vi "Semaphore.vi"() -> ()   [LabVIEW 2025]
panel:
  in  "Exit":bool
  in  "VISA resource name":refnum<visa-resource-name>
  in  "ON-OFF":bool
  in  "Enable ERROR Mod":bool
  in  "Timer ERROR":dbl
  in  "Timer ROSSO":dbl
  in  "Timer GIALLO":dbl
  in  "Timer VERDE":dbl
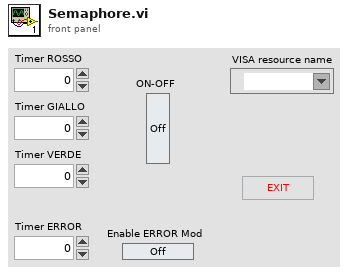
[diagram p1: front panel]
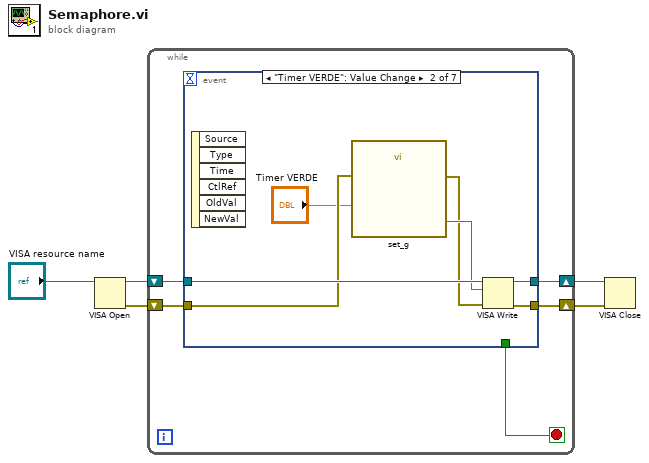
[diagram p0: block diagram]
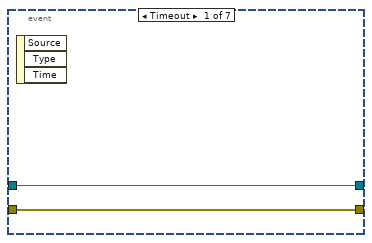
[diagram p2: hidden frame]
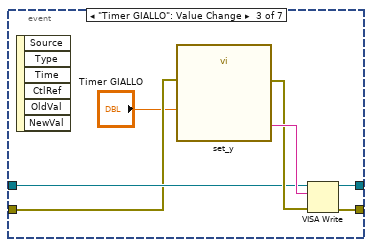
[diagram p3: hidden frame]
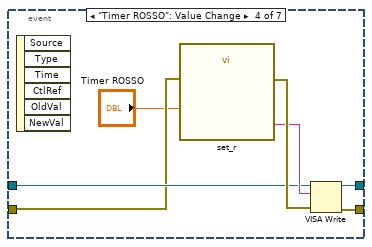
[diagram p4: hidden frame]
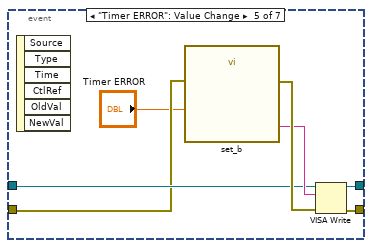
[diagram p5: hidden frame]
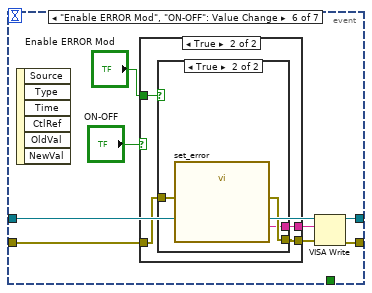
[diagram p6: hidden frame]
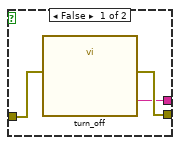
[diagram p7: hidden frame]
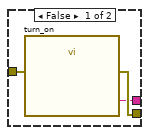
[diagram p8: hidden frame]
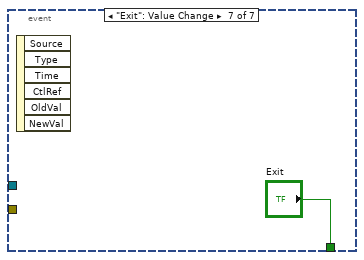
[diagram p9: hidden frame]
diagram:
  n1 = VISA Open(VISA resource name="VISA resource name") -> (VISA resource name=w3:refnum<visa-resource-name>, error out=w4:errorcluster)  [unwired: 4 in]
  n2 = while {
    shift-right: [w8] -> w2
    shift-left: w3 -> [w10]
    shift-right: [w7] -> w1
    shift-left: w4 -> [w9]
    stop <- w6 stop-if-true
    n3 = event shown="[1] \"Timer VERDE\": Value Change" {
      selector: _ -> [_ _ _ _ _ _ _]
      dyn-events: _ -> [_ _ _ _ _ _ _]
      timeout: _ -> [_ _ _ _ _ _ _]
      tunnel: w9 -> [w12 w16 w23 w30 w37 w44 _]
      tunnel: w10 -> [w11 w19 w24 w31 w38 w45 _]
      tunnel: [w11 w18 w22 w28 w35 w47 _] -> w8
      tunnel: [w12 w17 w21 w27 w34 w46 _] -> w7
      tunnel: [_ _ _ _ _ _ "Exit"] -> w6
      event Timeout {
        n4 = event-data() -> ()  [unwired: 1 in, 3 out]
      }
      event "Timer VERDE": Value Change {
        n5 = event-data() -> ()  [unwired: 1 in, 6 out]
        n6 = call "set_g"("timer"="Timer VERDE", "error in (no error)"=w16) -> ("Result"=w14:string, "error out"=w13:errorcluster)  [unwired: 12 in]
        n7 = VISA Write(VISA resource name=w19, write buffer=w14, error in (no error)=w13) -> (VISA resource name out=w18:refnum<visa-resource-name>, error out=w17:errorcluster)  [unwired: 1 out]
      }
      event "Timer GIALLO": Value Change {
        n8 = event-data() -> ()  [unwired: 1 in, 6 out]
        n9 = call "set_y"("timer"="Timer GIALLO", "error in (no error)"=w23) -> ("Result"=w26:string, "error out"=w25:errorcluster)  [unwired: 12 in]
        n10 = VISA Write(VISA resource name=w24, write buffer=w26, error in (no error)=w25) -> (VISA resource name out=w22:refnum<visa-resource-name>, error out=w21:errorcluster)  [unwired: 1 out]
      }
      event "Timer ROSSO": Value Change {
        n11 = event-data() -> ()  [unwired: 1 in, 6 out]
        n12 = call "set_r"("timer"="Timer ROSSO", "error in (no error)"=w30) -> ("Result"=w32:string, "error out"=w33:errorcluster)  [unwired: 12 in]
        n13 = VISA Write(VISA resource name=w31, write buffer=w32, error in (no error)=w33) -> (VISA resource name out=w28:refnum<visa-resource-name>, error out=w27:errorcluster)  [unwired: 1 out]
      }
      event "Timer ERROR": Value Change {
        n14 = event-data() -> ()  [unwired: 1 in, 6 out]
        n15 = call "set_b"("timer"="Timer ERROR", "error in (no error)"=w37) -> ("Result"=w39:string, "error out"=w40:errorcluster)  [unwired: 12 in]
        n16 = VISA Write(VISA resource name=w38, write buffer=w39, error in (no error)=w40) -> (VISA resource name out=w35:refnum<visa-resource-name>, error out=w34:errorcluster)  [unwired: 1 out]
      }
      event "Enable ERROR Mod", "ON-OFF": Value Change {
        n17 = event-data() -> ()  [unwired: 1 in, 6 out]
        n18 = case shown="True" "ON-OFF" {
          tunnel: w44 -> [w51 w54]
          tunnel: [w50 w53] -> w43
          tunnel: [w49 w52] -> w42
          tunnel: "Enable ERROR Mod" -> [_ w55]
          frame False {
            n19 = call "turn_off"("error in (no error)"=w51) -> ("Result"=w49:string, "error out"=w50:errorcluster)  [unwired: 13 in]
          }
          frame True {
            n20 = case shown="True" w55 {
              tunnel: w54 -> [w58 w61]
              tunnel: [w57 w60] -> w53
              tunnel: [w56 w59] -> w52
              frame False {
                n21 = call "turn_on"("error in (no error)"=w58) -> ("Result"=w56:string, "error out"=w57:errorcluster)  [unwired: 13 in]
              }
              frame True {
                n22 = call "set_error"("error in (no error)"=w61) -> ("Result"=w59:string, "error out"=w60:errorcluster)  [unwired: 13 in]
              }
            }
          }
        }
        n23 = VISA Write(VISA resource name=w45, write buffer=w42, error in (no error)=w43) -> (VISA resource name out=w47:refnum<visa-resource-name>, error out=w46:errorcluster)  [unwired: 1 out]
      }
      event "Exit": Value Change {
        n24 = event-data() -> ()  [unwired: 1 in, 6 out]
      }
    }
  }
  n25 = VISA Close(VISA resource name=w2, error in (no error)=w1) -> ()  [unwired: 1 out]
